vi "Launch Nested Actors.vi"(8 "error in (no error)":errorcluster, 11 "Cylinder in":refnum<class "Cylinder.lvclass">) -> (0 "error out":errorcluster, 3 "Cylinder out":refnum<class "Cylinder.lvclass">)   [LabVIEW 2015, in "cRIO-Carbondioxide.lvlib" / "CO2-Actor.lvlib" / "Cylinder.lvclass"]
uses:
  Cylinder.lvclass
  Cylinder.lvclass/Cylinder.ctl
  Valve/Action.ctl
  CO2 Actor/CO2 Actor.lvclass
  Valve/Valve.lvclass
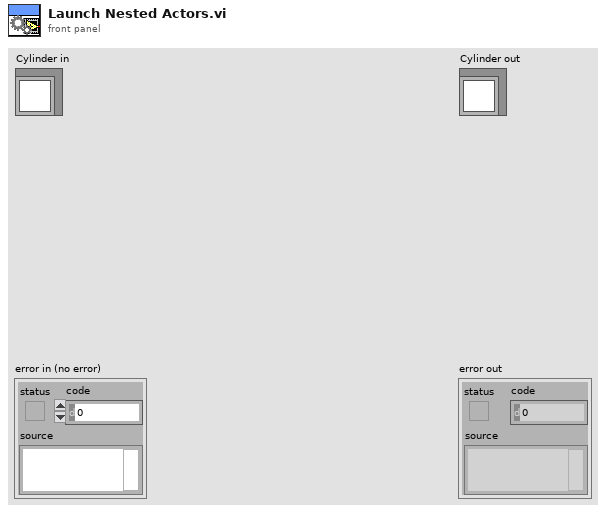
[diagram p1: front panel]
types:
  T1 = typedef "Action.ctl" = enum16{"Open", "Close", "None"}
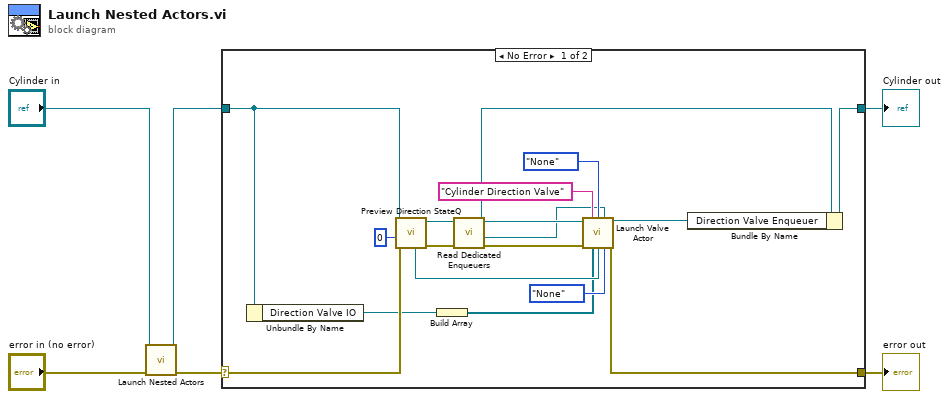
[diagram p0: block diagram]
diagram:
  n1 = call-parent "Launch Nested Actors.vi"("error in (no error)"="error in (no error)", "CO2 Actor in"="Cylinder in") -> ("error out"=w3:errorcluster, "CO2 Actor out"=w1:refnum<class "Cylinder.lvclass">)  [unwired: 8 in]
  n2 = case shown="No Error" w3 {
    selector: w3 -> [w16 w25]
    tunnel: [w23 w25] -> w6
    tunnel: [w21 w24] -> w5
    tunnel: w1 -> [w9 w24]
    frame No Error {
      n3 = Unbundle By Name(w9) -> ("Direction Valve IO"=w8:refnum<k21>)
      n4 = call "Preview Direction StateQ.vi"("error in (no error)"=w16, "timeout in ms (-1)"=0, "Cylinder in"=w9) -> ("error out"=w14:errorcluster, "Cylinder out"=w12:refnum<class "Cylinder.lvclass">, "Valve StateQ"=w15:refnum<queue>)  [unwired: 4 in, 2 out]
      n5 = Build Array(w8) -> (w7:refnum<k21>[])
      n6 = call "Read Dedicated Enqueuers.vi"("error in (no error)"=w14, "CO2 Actor in"=w12) -> ("error out"=w13:errorcluster, "DedicatedEnQrs"=w10:refnum<queue>, "CO2 Actor out"=w11:refnum<class "Cylinder.lvclass">)  [unwired: 6 in, 1 out]
      n7 = call "Launch Valve Actor.vi"("Caller Actor in"=w11, "Name"="Cylinder Direction Valve", "Start Action (Open)"=Action."None", "DedicatedEnQrs"=w10, "error in (no error)"=w13, "SHV"=w7, "StateQ"=w15, "Stop Action (Close)"=Action."None") -> ("Caller-To-Actor Enqueuer"=w20:refnum<class "Message Enqueuer.lvclass">, "error out"=w23:errorcluster)  [unwired: 6 in]
      n8 = Bundle By Name(cluster=w11, "Direction Valve Enqueuer"=w20) -> (w21:refnum<class "Cylinder.lvclass">)
    }
    frame Error {
    }
  }
  "error out" <- w6
  "Cylinder out" <- w5
